vi "initialize cipher.vi"(5 "encrypt?":bool, 7 "IV":string, 8 "error in":errorcluster, 9 "key":string, 10 "cipher name":string, 11 "lvlibcrypto digest in":refnum<class "lvlibcrypto cipher.lvclass">) -> (0 "error out":errorcluster, 2 "sizes":T1, 3 "lvlibcrypto digest out":refnum<class "lvlibcrypto cipher.lvclass">)   [LabVIEW 2016, in "lvlibcrypto cipher.lvclass"]
uses:
  lvlibcrypto cipher.lvclass
  lvlibcrypto cipher.lvclass/lvlibcrypto cipher.ctl
  add all ciphers.vi
  lv tls dll.lvlib
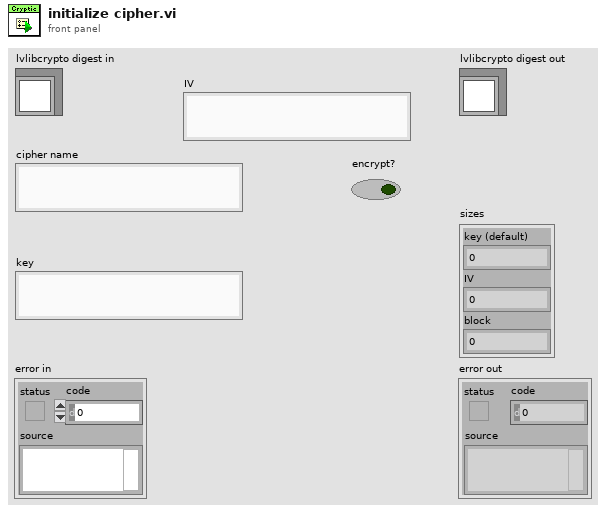
[diagram p1: front panel]
types:
  T1 = cluster{"key (default)":i32, "IV":i32, "block":i32}
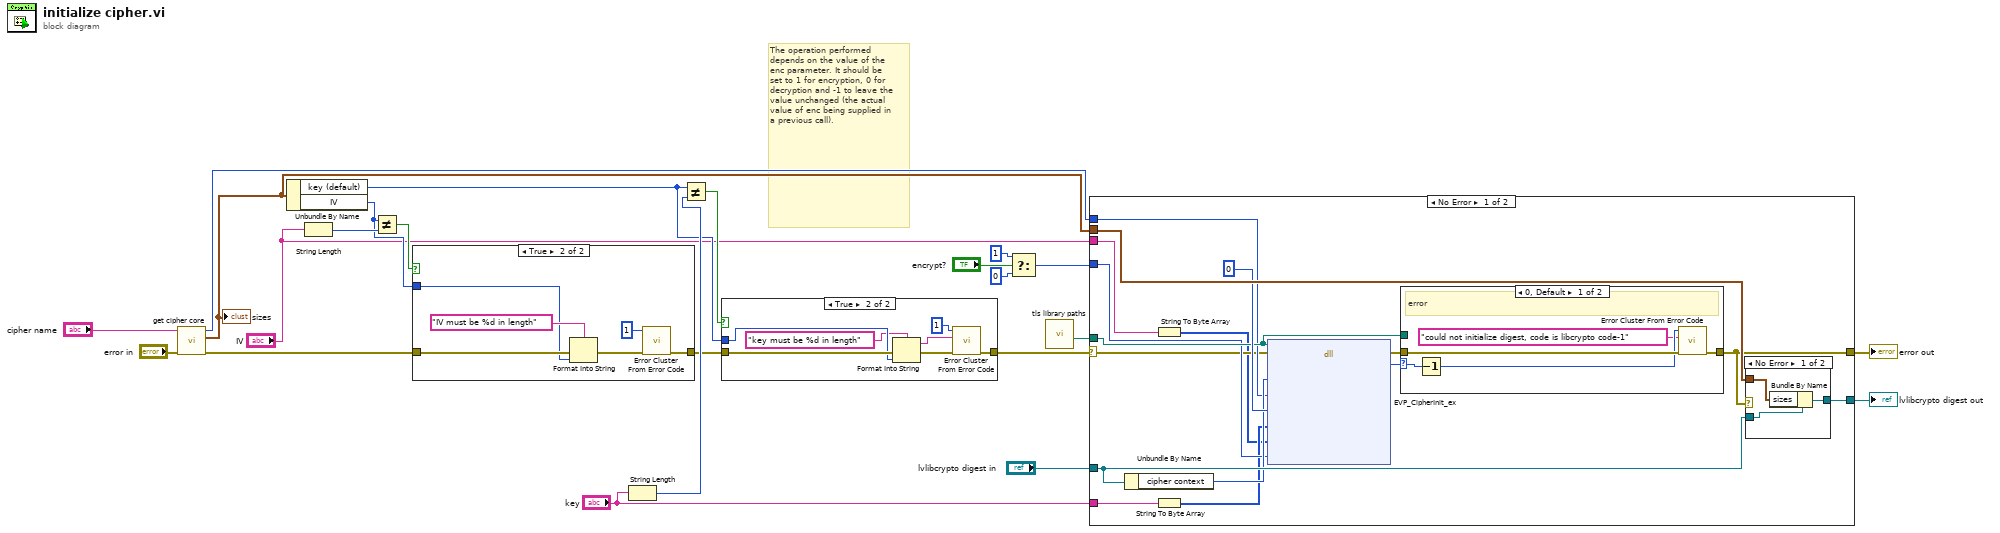
[diagram p0: block diagram]
diagram:
  # "The operation performed depends on the value of the enc parameter. It should be set to 1 for encryption, 0 for decryption and -1 to leave the value unchanged (the actual value of enc being supplied in a previous call)."
  n1 = call "get cipher core.vi"("error in"="error in", "cipher name"="cipher name") -> ("error out"=w17:errorcluster, "sizes"=w11:T1, "cipher"=w14:u64)  [unwired: 7 in]
  "sizes" <- w11
  n2 = Unbundle By Name(w11) -> ("key (default)"=w3:i32, "IV"=w4:i32)
  n3 = String Length(string="IV") -> (length=w10:i32)
  n4 = Not Equal?(x=w4, y=w10) -> (x != y?=w5:bool)
  n5 = case shown="True" w5 {
    tunnel: w17 -> [w24 w30]
    tunnel: [w24 w29] -> w8
    tunnel: w4 -> [_ w25]
    frame False {
    }
    frame True {
      n6 = Format Into String(format string="IV must be %d in length", error in=w30, w25) -> (error out=w27:errorcluster)  [unwired: 1 in, 1 out]
      n7 = call <vilib>:"Error Cluster From Error Code.vi"("error in (no error)"=w27, "error code (0)"=1) -> ("error out"=w29:errorcluster)  [unwired: 7 in]
    }
  }
  n8 = String Length(string="key") -> (length=w9:i32)
  n9 = Not Equal?(x=w3, y=w9) -> (x != y?=w6:bool)
  n10 = case shown="True" w6 {
    tunnel: w8 -> [w31 w38]
    tunnel: [w31 w37] -> w7
    tunnel: w3 -> [_ w36]
    frame False {
    }
    frame True {
      n11 = Format Into String(format string="key must be %d in length", error in=w38, w36) -> (resulting string=w34:string, error out=w35:errorcluster)  [unwired: 1 in]
      n12 = call <vilib>:"Error Cluster From Error Code.vi"("error in (no error)"=w35, "error message (\"\")"=w34, "error code (0)"=1) -> ("error out"=w37:errorcluster)  [unwired: 6 in]
    }
  }
  n13 = Select(t=1, s="encrypt?", f=0 ("t")) -> (s? t:f=w13:i32)
  n14 = call "tls library paths.vi"() -> ("libcrypto"=w12:path)  [unwired: 8 in, 3 out]
  n15 = case shown="No Error" w7 {
    selector: w7 -> [w44 w65]
    tunnel: [w53 w66] -> w19
    tunnel: "lvlibcrypto digest in" -> [w54 w66]
    tunnel: [w43 w65] -> w16
    tunnel: w14 -> [w45 _]
    tunnel: w11 -> [w52 _]
    tunnel: w13 -> [w46 _]
    tunnel: w12 -> [w48 _]
    tunnel: "key" -> [w42 _]
    tunnel: "IV" -> [w39 _]
    frame No Error {
      n16 = Unbundle By Name(w54) -> ("cipher context"=w47:u64)
      n17 = String To Byte Array(string=w39) -> (unsigned byte array=w40:u8[])
      n18 = String To Byte Array(string=w42) -> (unsigned byte array=w41:u8[])
      n19 = dll-call lib="C:/Users/IEUser/Desktop/tlssimple/libcrypto-41.dll" fn="EVP_CipherInit_ex"(path in=w48, error in=w44, "context"=w47, "cipher type"=w45, "engine null"=u64 0, "key"=w41, "IV"=w40, "encode or decode"=w46) -> (error out=w49:errorcluster, "ret"=w50:i32)  [unwired: 7 in, 1 out]
      n20 = case shown="0, Default" w50 {
        selector: w50 -> [w57 _]
        tunnel: [w58 w60] -> w43
        tunnel: w49 -> [w59 w60]
        tunnel: w48 -> [_ _]
        frame 0, Default {
          # "error"
          n21 = Decrement(x=w57) -> (x-1=w56:i32)
          n22 = call <vilib>:"Error Cluster From Error Code.vi"("error in (no error)"=w59, "error message (\"\")"="could not initialize digest, code is libcrypto code-1" ("error message (\"\")"), "error code (0)"=w56) -> ("error out"=w58:errorcluster)  [unwired: 6 in]
        }
        frame 1 {
          # "success"
        }
      }
      n23 = case shown="No Error" w43 {
        tunnel: w54 -> [w63 w64]
        tunnel: [w62 w64] -> w53
        tunnel: w52 -> [w61 _]
        frame No Error {
          n24 = Bundle By Name(cluster=w63, "sizes"=w61) -> (w62:refnum<class "lvlibcrypto cipher.lvclass">)
        }
        frame Error {
        }
      }
    }
    frame Error {
    }
  }
  "error out" <- w16
  "lvlibcrypto digest out" <- w19
